vi "Cell I Readback.vi"(7 "Box ID":u8, 8 "error in (no error)":errorcluster, 10 "Channel":u16=1 min=1 max=12 step=1, 11 "BS120x in":refnum<class "BS120x.lvclass">) -> (0 "error out":errorcluster, 2 "Current (mA)":dbl, 3 "BS120x out":refnum<class "BS120x.lvclass">)   [LabVIEW 2021, in "BS120x Driver.lvlib" / "BS120x.lvclass"]
doc: "Returns the current of the specified Battery Simulator 1200 cell.\n(c) 2019 Bloomy Controls, Inc. All rights reserved."
uses:
  BS120x.lvclass
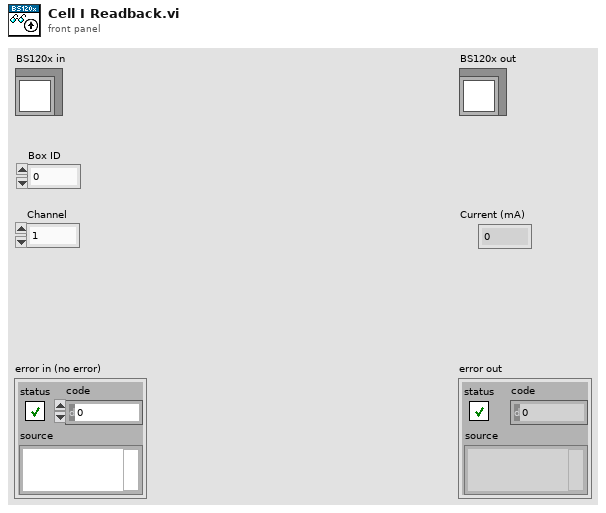
[diagram p1: front panel]
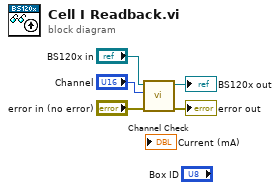
[diagram p0: block diagram]
diagram:
  n1 = call "Channel Check.vi"("error in (no error)"="error in (no error)", "Channel"="Channel", "BS120x in"="BS120x in") -> ("error out"=→"error out":errorcluster, "BS120x out"=→"BS120x out":refnum<class "BS120x.lvclass">)  [unwired: 7 in]
